vi "Create.vi"(8 "error in (no error)":errorcluster, 10 "Input":string) -> (0 "error out":errorcluster, 3 "Proto":refnum<class "Proto.lvclass">)   [LabVIEW 2020, in "Proto.lvclass"]
uses:
  Proto.lvclass
  Helpers/Helpers.lvlib
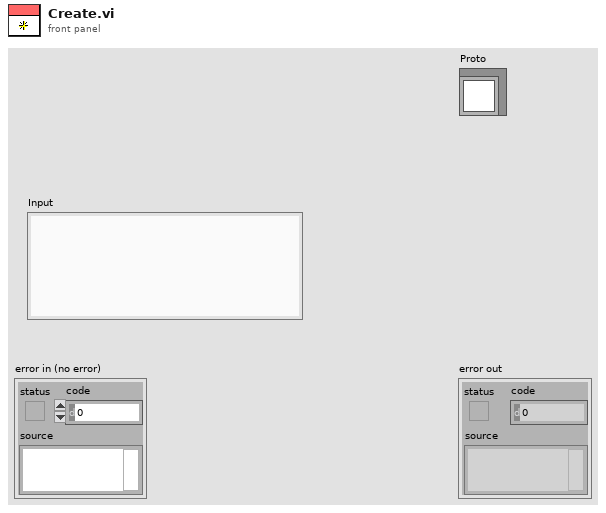
[diagram p1: front panel]
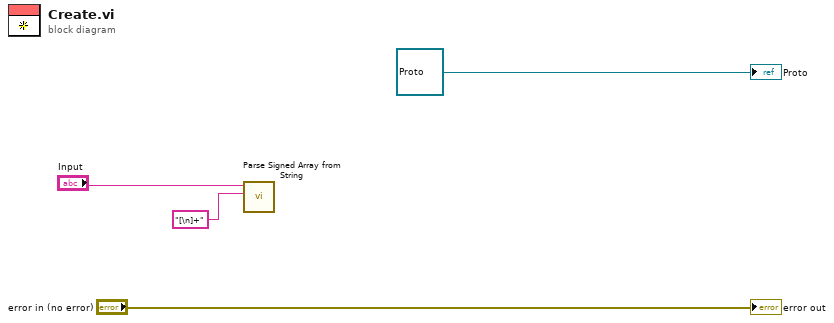
[diagram p0: block diagram]
diagram:
  n1 = call "Parse Signed Array from String.vi"("Delimiter regex"="[\n]+", "Input"="Input") -> ()  [unwired: 8 in, 2 out]
  "error out" <- "error in (no error)"
  "Proto" <- refnum<class "Proto.lvclass"> refnum ("Proto")
